vi "F Dwf Analog Out Node Function Set.vi"(7 "func":u8, 8 "error in (no error)":errorcluster, 9 "node":i32, 10 "idxChannel":i32, 11 "hdwf":i32) -> (0 "error out":errorcluster, 3 "function return":i32)   [LabVIEW 2019, in "Olasdwf.lvlib"]
doc: "DWFAPI int FDwfAnalogOutNodeFunctionInfo(HDWF hdwf, int idxChannel, AnalogOutNode node, int *pfsfunc); DWFAPI int FDwfAnalogOutNodeFunctionSet(HDWF hdwf, int idxChannel, AnalogOutNode node, FUNC func);"
uses:
  Olasdwf.lvlib
  Windows/System32/dwf.dll
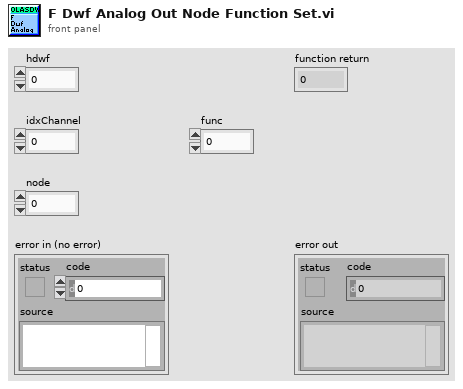
[diagram p1: front panel]
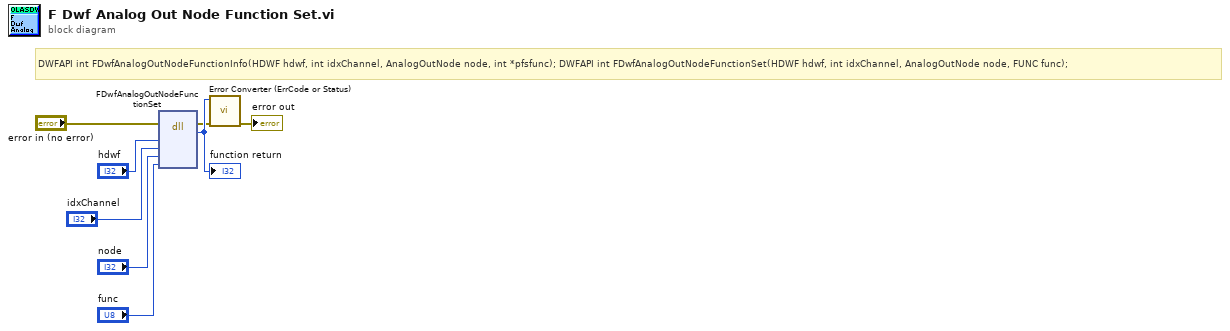
[diagram p0: block diagram]
diagram:
  # "DWFAPI int FDwfAnalogOutNodeFunctionInfo(HDWF hdwf, int idxChannel, AnalogOutNode node, int *pfsfunc); DWFAPI int FDwfAnalogOutNodeFunctionSet(HDWF hdwf, int idxChannel, AnalogOutNode node, FUNC func);"
  n1 = dll-call lib="C:/Windows/System32/dwf.*" fn="FDwfAnalogOutNodeFunctionSet"(error in="error in (no error)", "hdwf"="hdwf", "idxChannel"="idxChannel", "node"="node", "func"="func") -> (error out=w2:errorcluster, w8:i32)  [unwired: 6 in, 1 out]
  "function return" <- w8
  n2 = call "Error Converter (ErrCode or Status).vi"("error in (no error)"=w2, "error code"=w8) -> ("error out"=→"error out":errorcluster)  [unwired: 9 in]
